vi "UT_Cognex.vi"() -> ()   [LabVIEW 2019, in "Kolmogan Library 1.lvlib"]
uses:
  Kolmogan Library 1.lvlib
panel:
  out "current time 5":timestamp
  out "指示燈":bool
  out "current time":timestamp
  out "Data":string
  out "Final result":string
  out "Trigger Success":bool
  out "螺絲檢測結果":string="檢測完成"
  out "右邊結果":string
  out "左邊結果":string
  out "檢測結果R":bool
  out "檢測結果L":bool
  out "R array":sgl[][](array[numeric])
  out "L array":sgl[][](array[numeric])
  out "掃高度次數":i32
  out "End time 4":timestamp=timestamp(3742957067.58093 s since 1904-01-01)
  out "移動完成 4":bool=TRUE
  out "Error status 4":bool
  out "等候逾時 4":bool
  out "剩餘秒數 4":i32=5
  in  "等候秒數 4":i32=40
  out "current time 4":timestamp=timestamp(3742957049.546739 s since 1904-01-01)
  out "找到原點":bool=TRUE
  in  "Trigger":u16(ring) items=["等待觸發", "觸發拍攝"]
  out "current time 3":timestamp=timestamp(3742956976.4306865 s since 1904-01-01)
  out "剩餘秒數 3":i32=9
  out "等候逾時 3":bool
  out "Error status 3":bool
  out "移動完成 3":bool=TRUE
  out "Motion State":bool[](array[boolean])=[FALSE, TRUE, TRUE, FALSE, FALSE, FALSE, FALSE, FALSE, FALSE, FALSE, FALSE, TRUE, FALSE, FALSE, FALSE, TRUE, FALSE, FALSE, FALSE, FALSE, FALSE, FALSE, FALSE, FALSE, FALSE, FALSE, FALSE, FALSE, FALSE, FALSE, FALSE, FALSE]
  in  "等候秒數 3":i32=15
  out "current time 2":timestamp=timestamp(3742956973.4187617 s since 1904-01-01)
  out "Error status 2":bool
  out "等候逾時 2":bool
  out "剩餘秒數 2":i32=5
  in  "等候秒數 2":i32=15
  out "State machine":i32=4
  out "等待觸發":bool=TRUE
  out "Offset array":dbl[](array[numeric])
  out "分析計算delay":u32=100
  out "使用流程":bool
  out "螺絲高度LL":dbl=2.1 format="%#_13g"
  out "螺絲高度UL":dbl=2.4009
  out "txt path":path
  out "L_file":string
  out "R_file":string
  in  "D2502.1 螺絲檢測 Ready":bool=TRUE
  in  "D2610 螺絲檢測完成":i16
  out "error out 2":errorcluster
  out "指令結果":string
  out "等待指令":string
  out "密碼":string
  out "帳號":string
  out "error out":errorcluster
  out "Success":bool
  in  "選項二: 觸發":bool
  in  "選項一: 監聽結果":bool
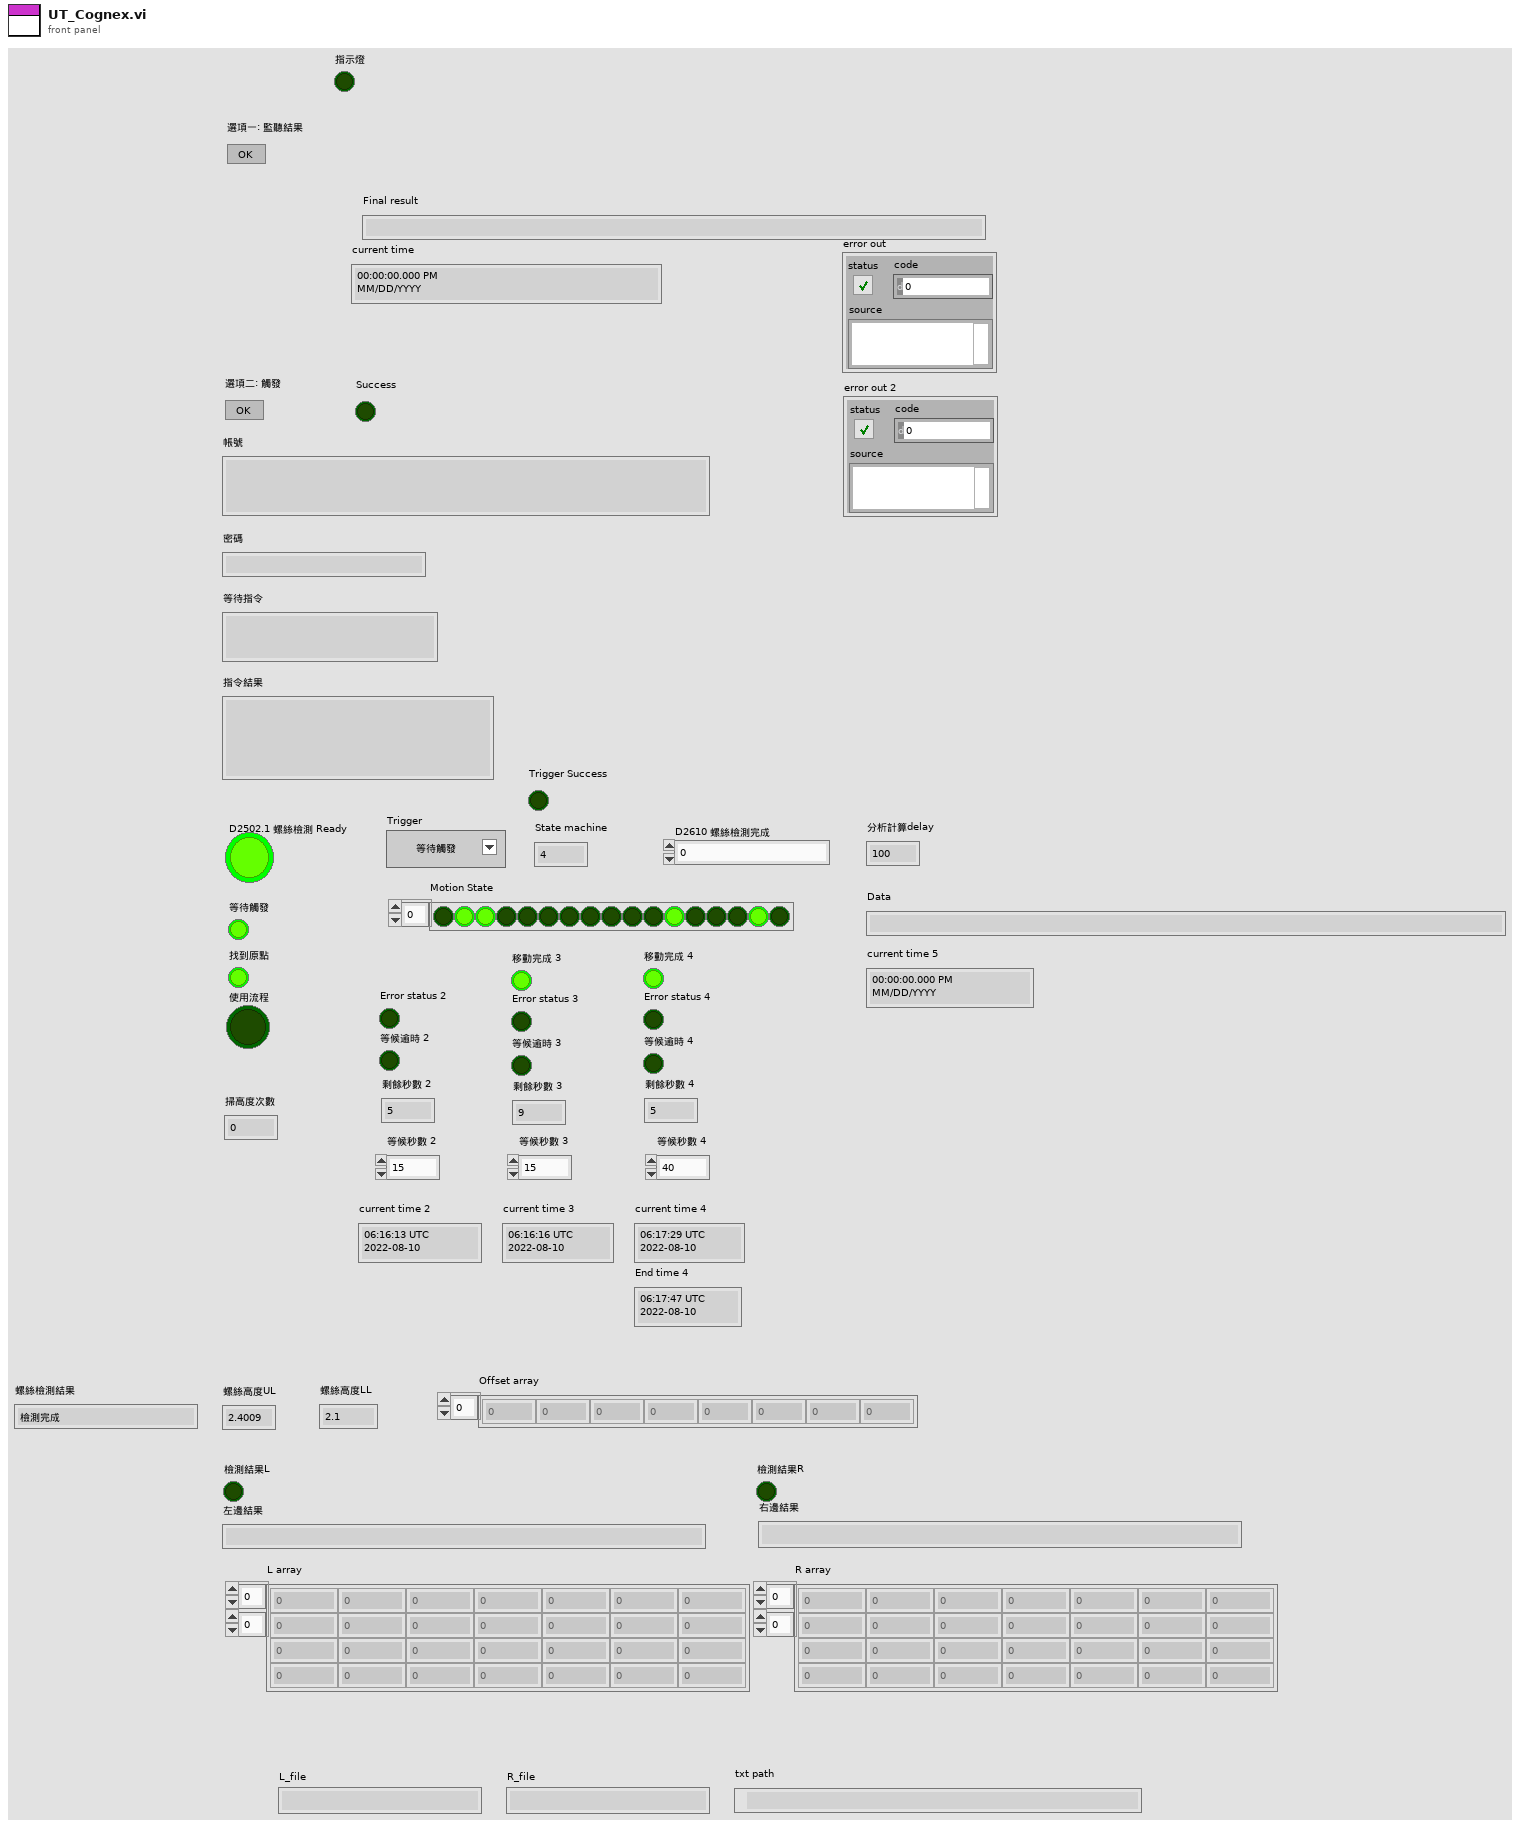
[diagram p1: front panel]
types:
  T1 = cluster{"sh_1":dbl, "sh_2":dbl, "sh_3":dbl, "sh_4":dbl, "sh_5":dbl, "sh_6":dbl}
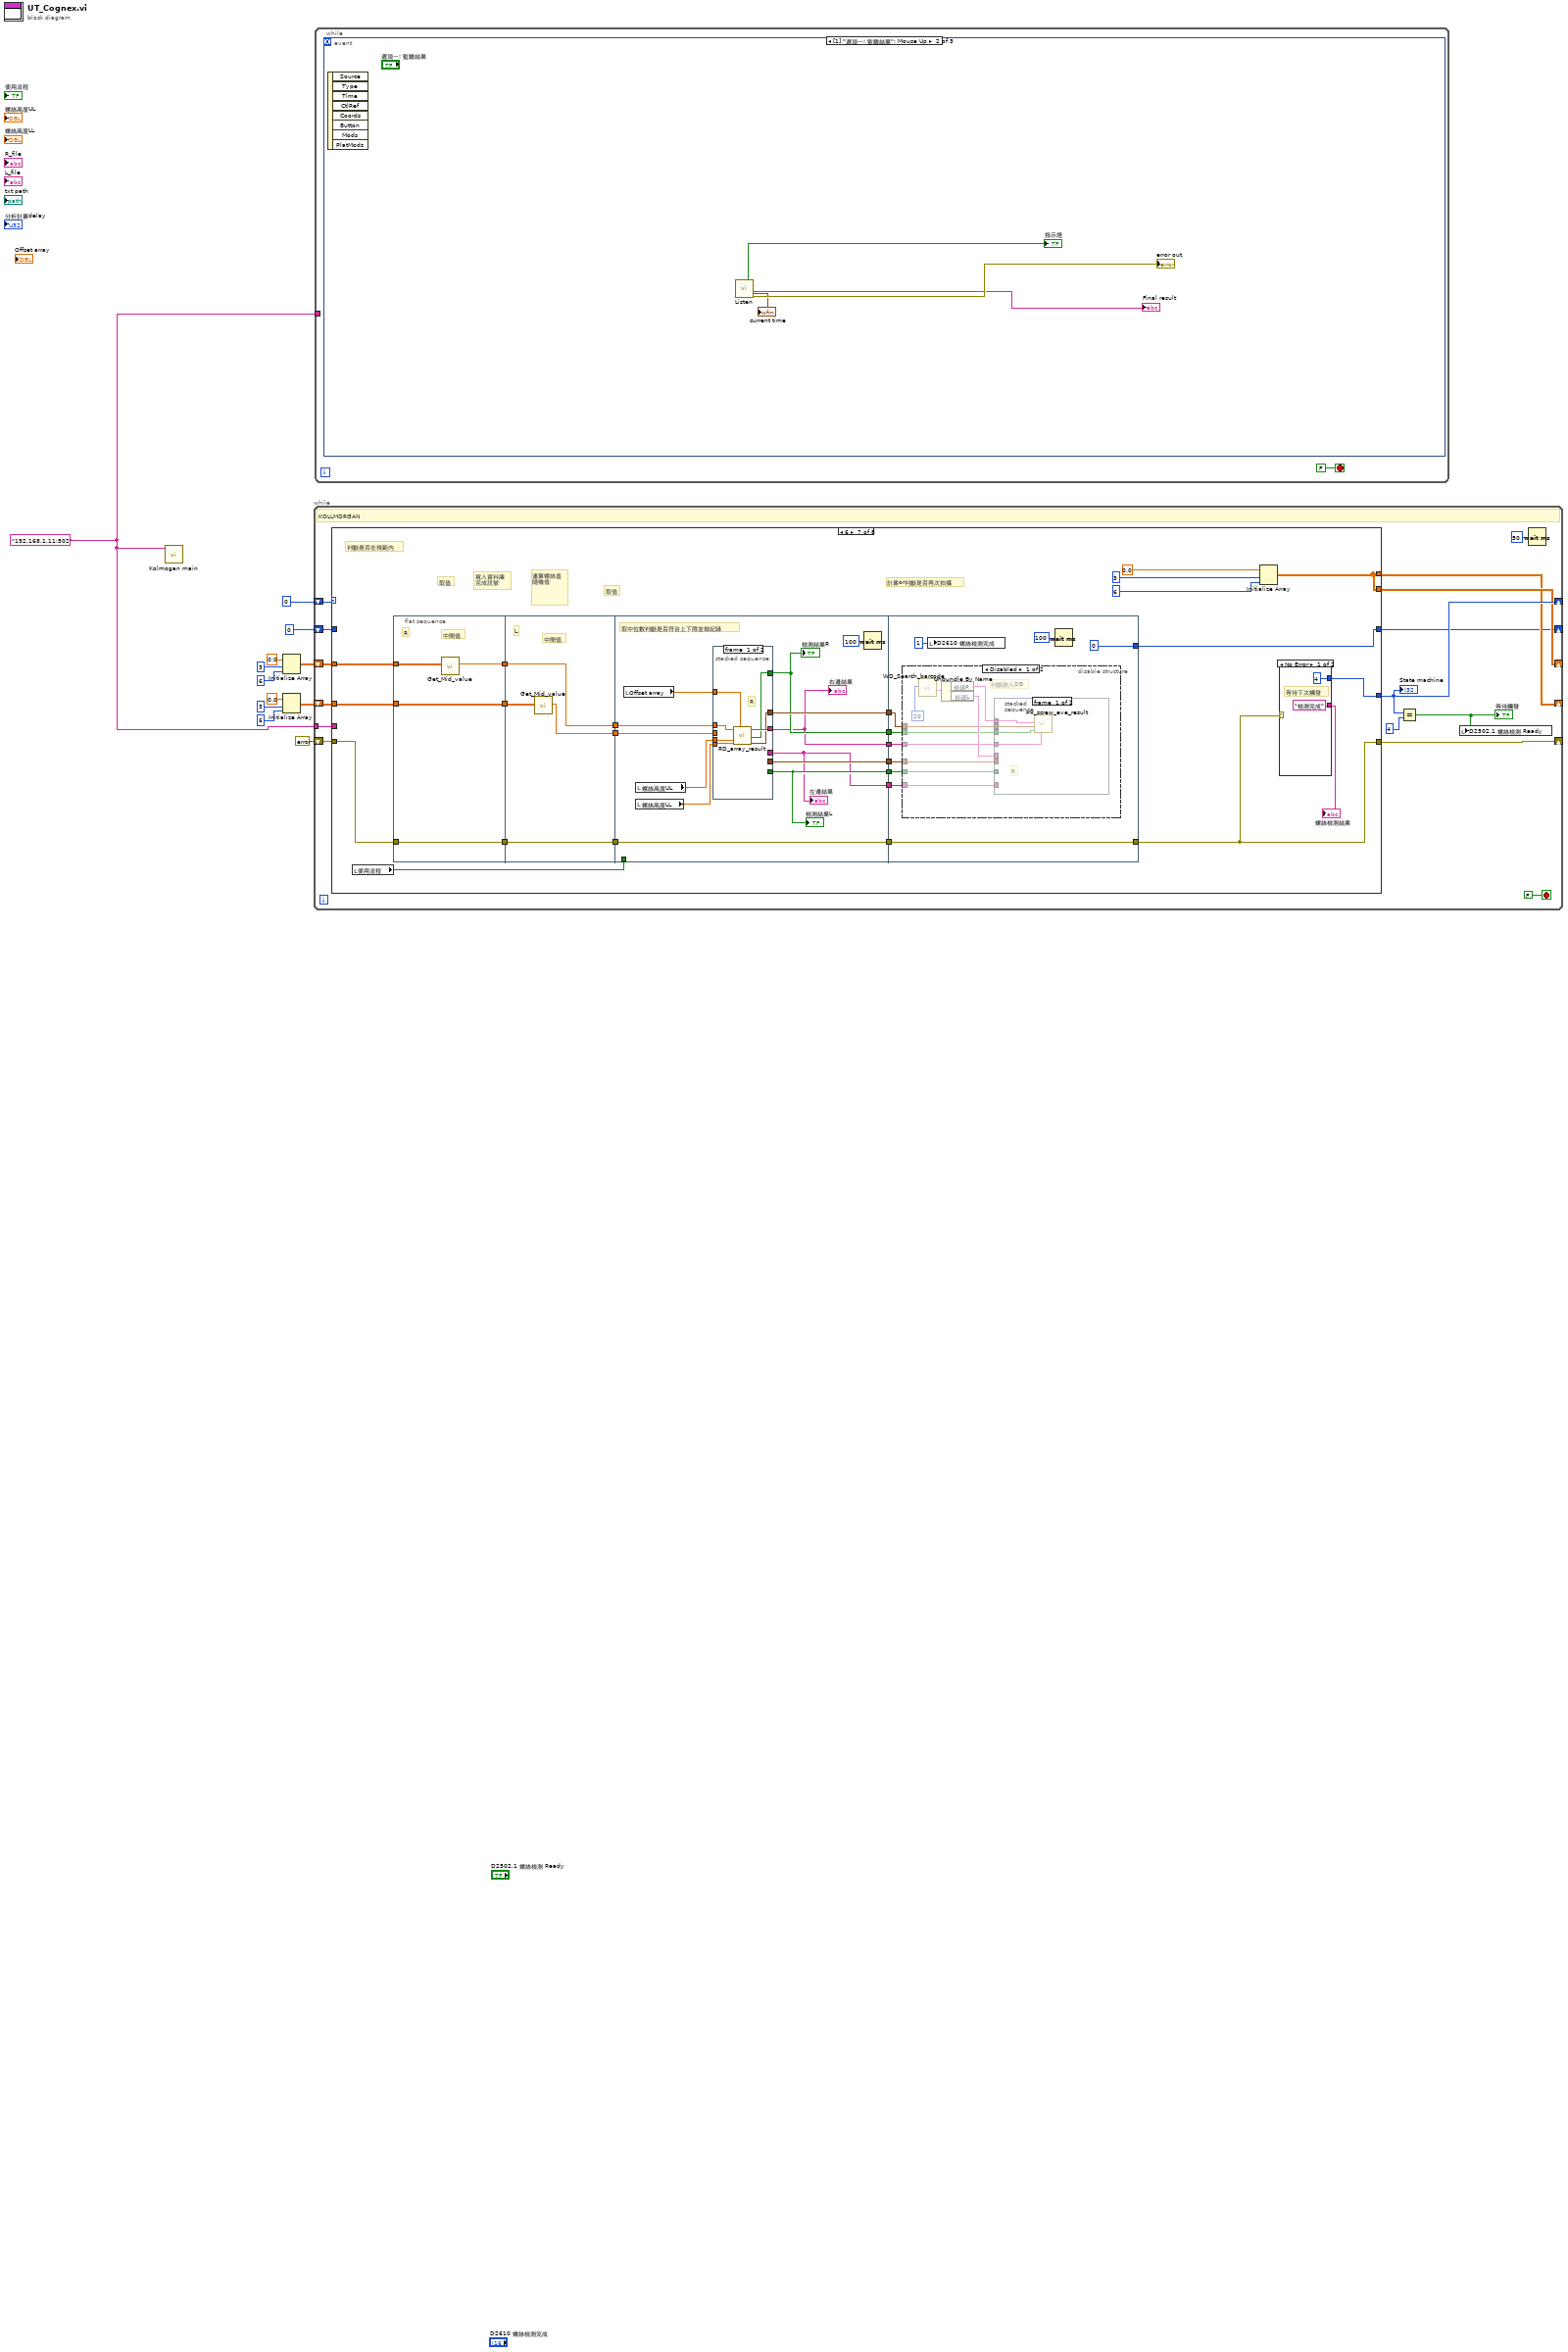
[diagram p0: block diagram]
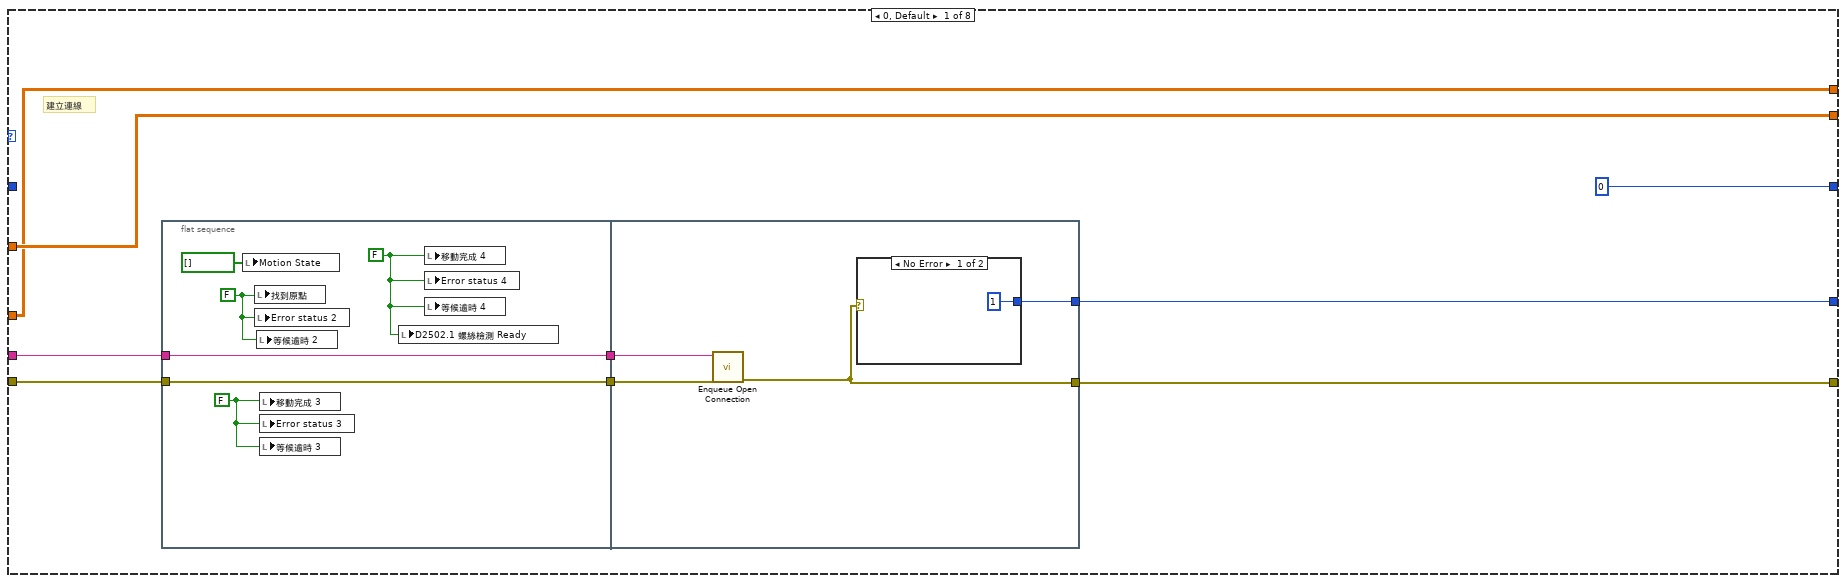
[diagram p2: hidden frame]
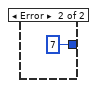
[diagram p3: hidden frame]
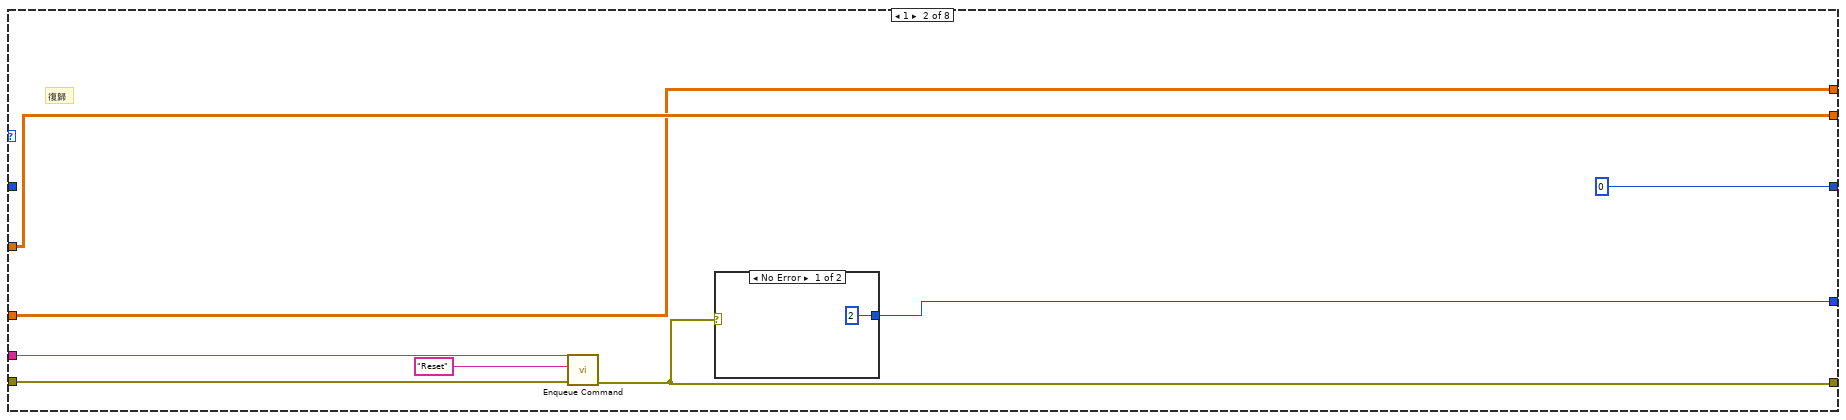
[diagram p4: hidden frame]
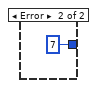
[diagram p5: hidden frame]
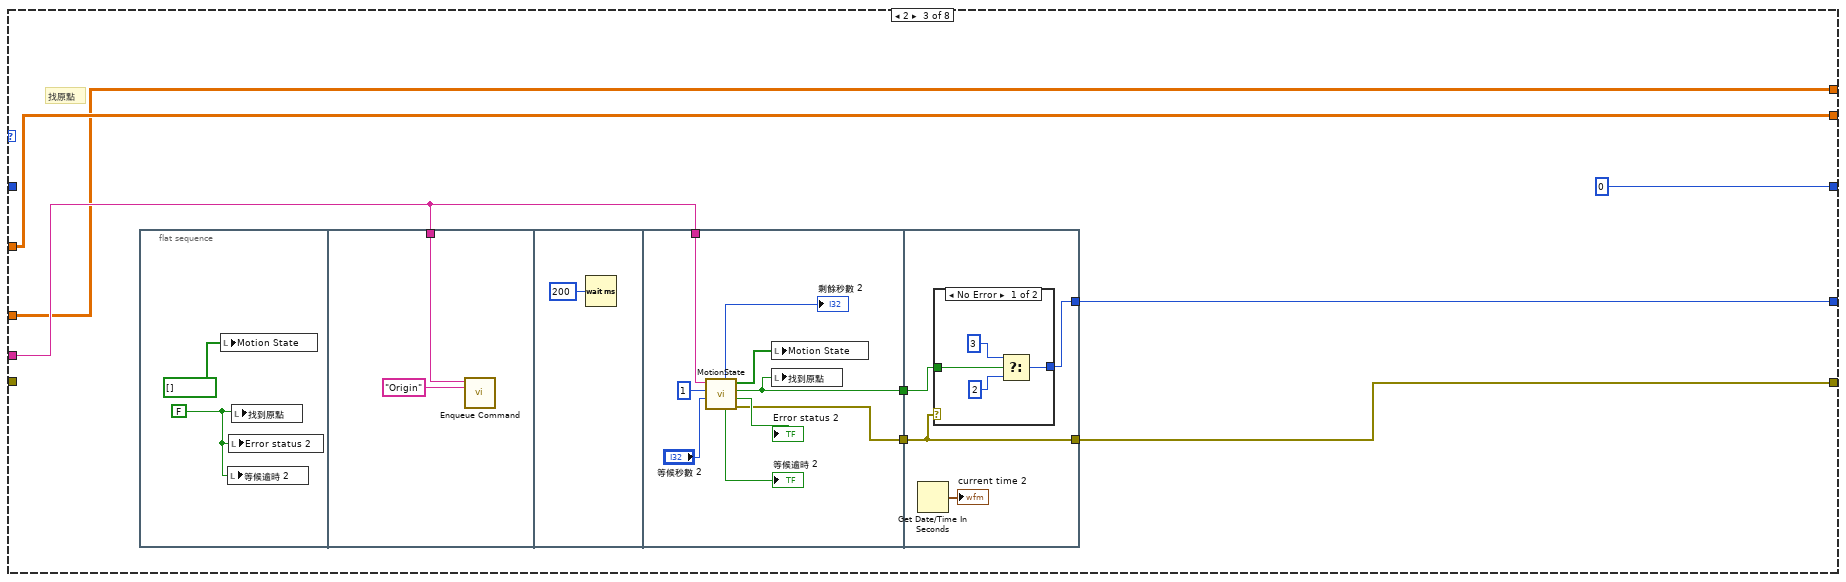
[diagram p6: hidden frame]
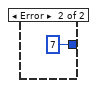
[diagram p7: hidden frame]
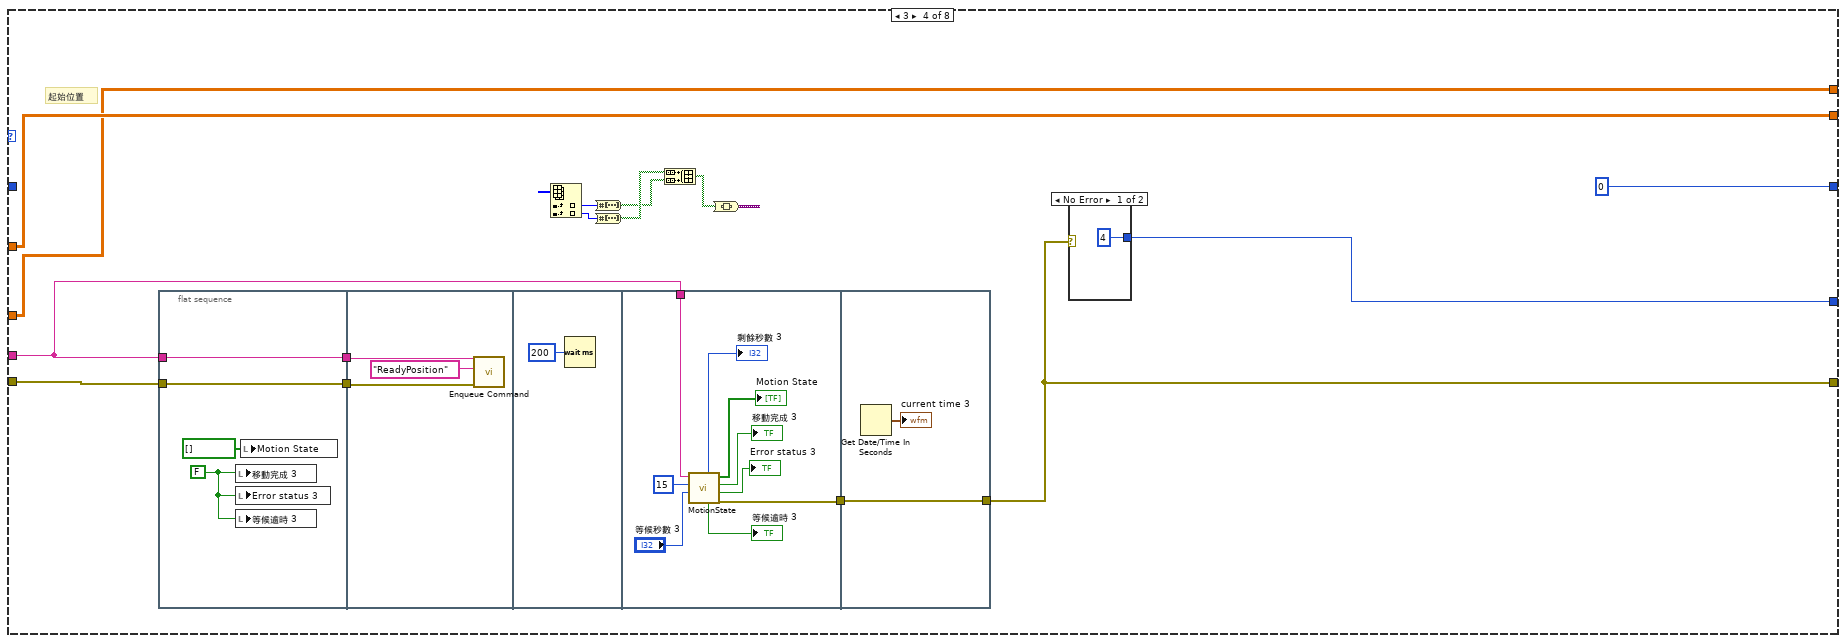
[diagram p8: hidden frame]
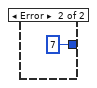
[diagram p9: hidden frame]
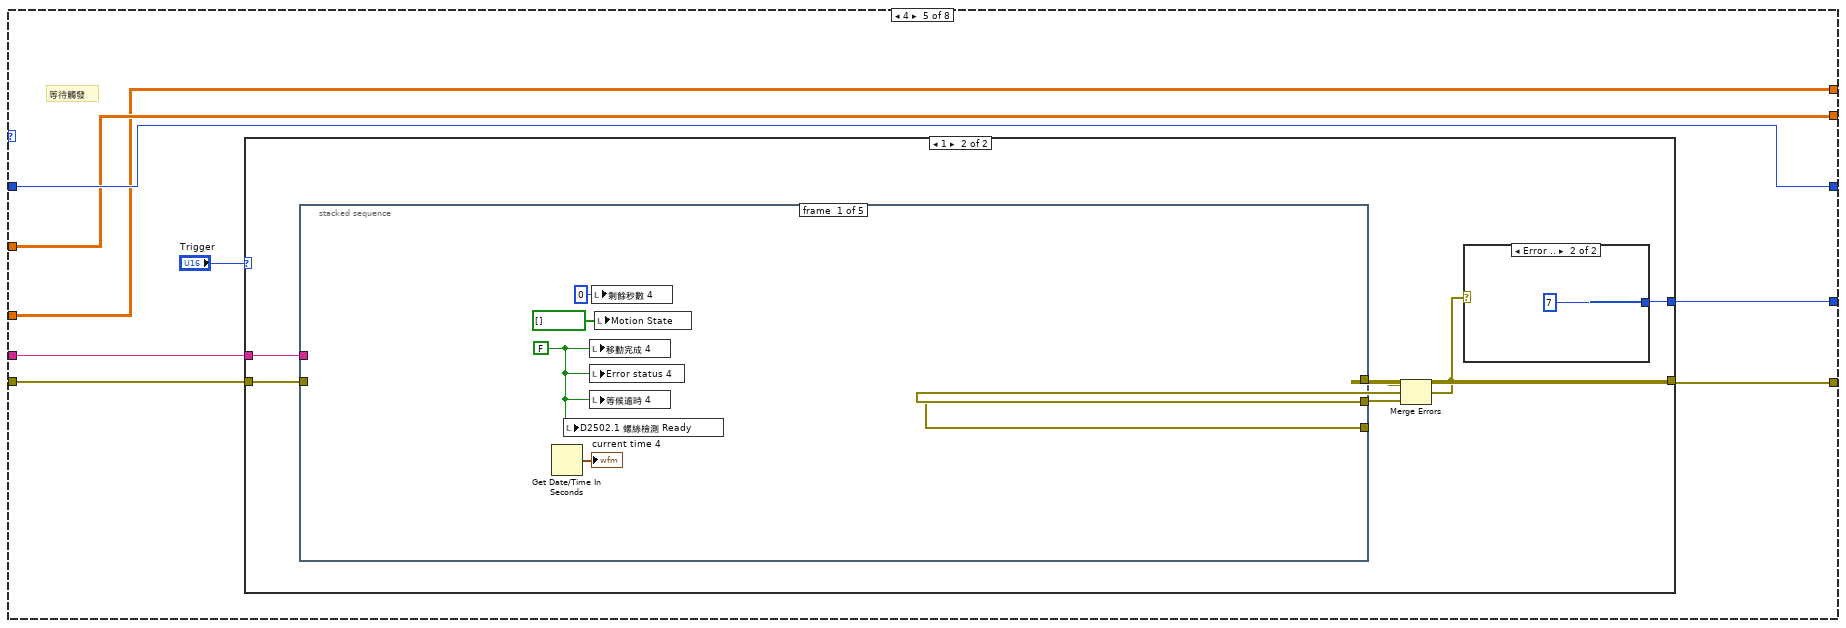
[diagram p10: hidden frame]
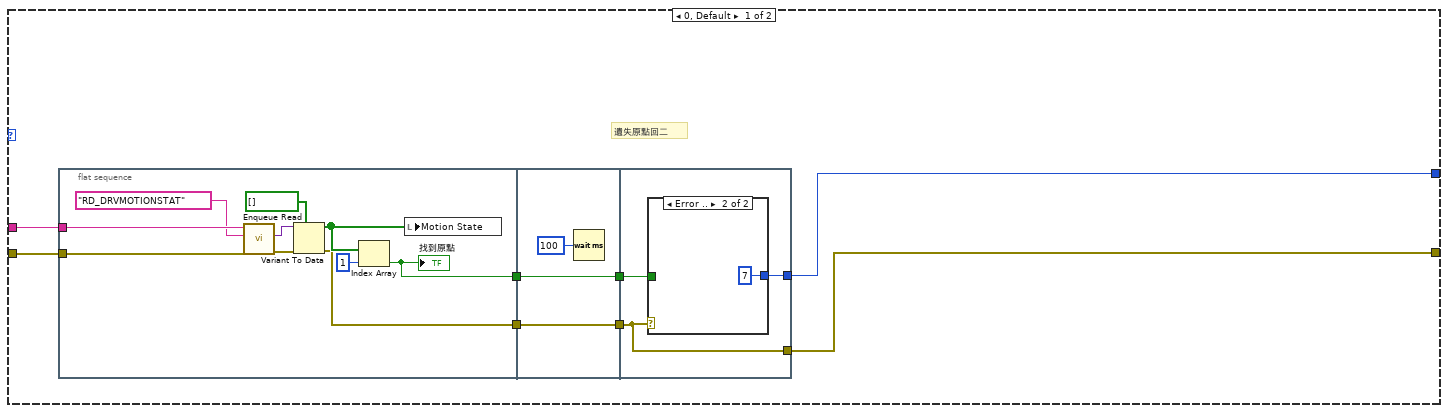
[diagram p11: hidden frame]
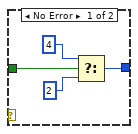
[diagram p12: hidden frame]
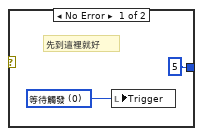
[diagram p13: hidden frame]
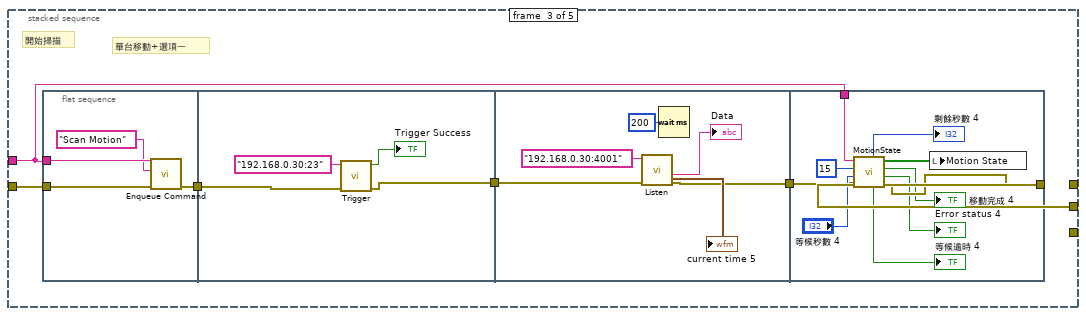
[diagram p15: hidden frame]
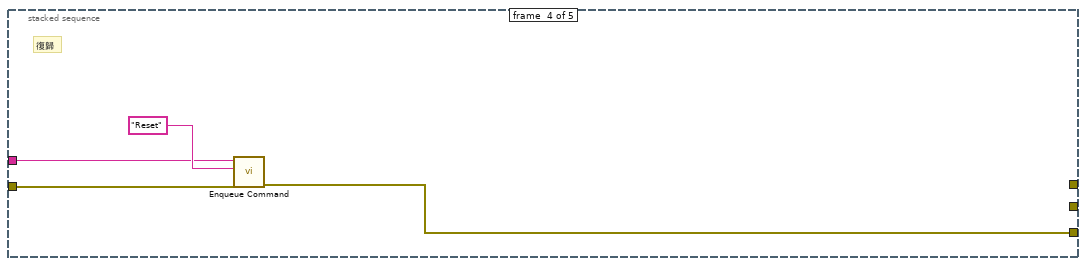
[diagram p16: hidden frame]
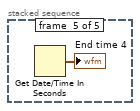
[diagram p17: hidden frame]
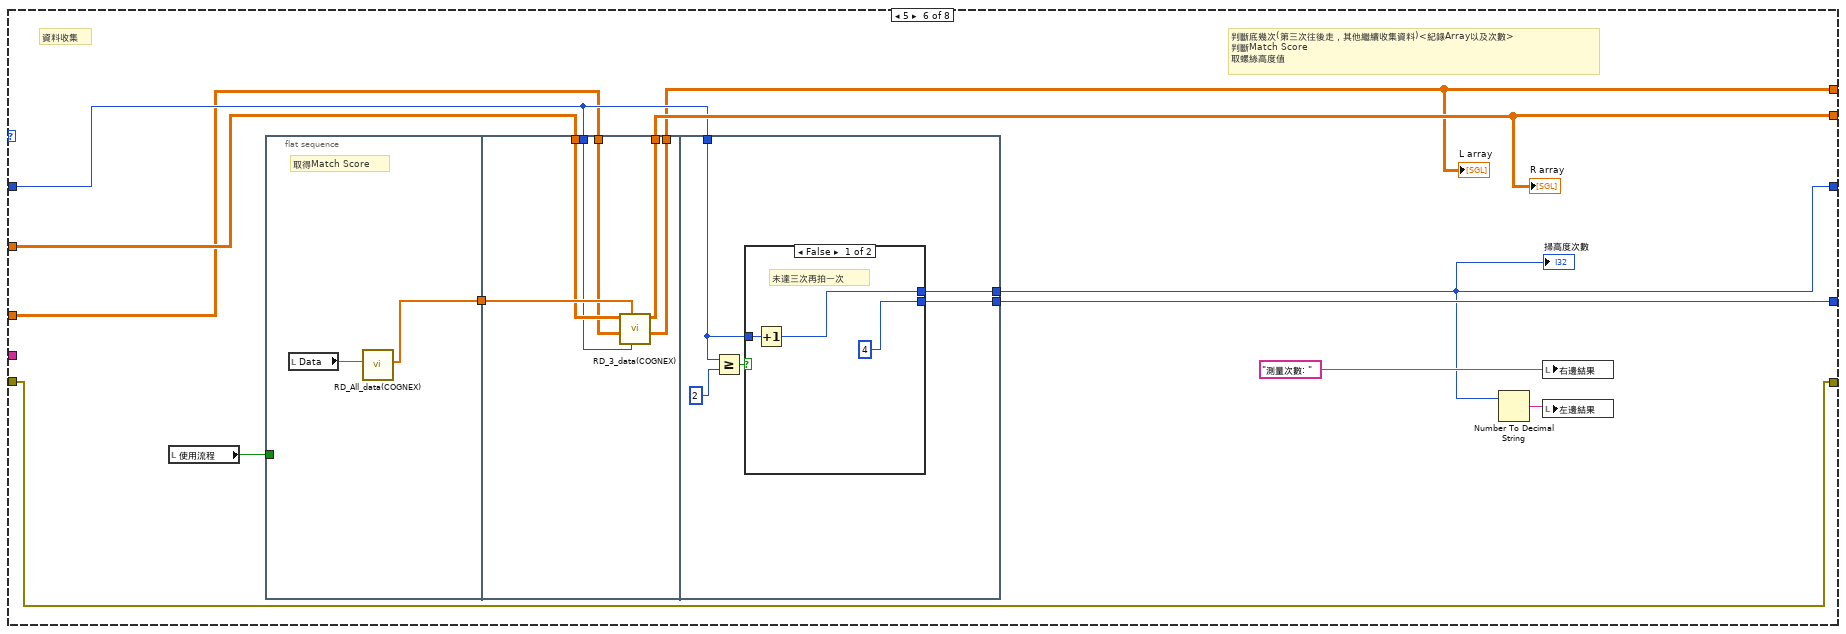
[diagram p18: hidden frame]
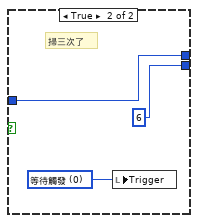
[diagram p19: hidden frame]
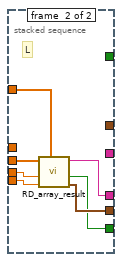
[diagram p20: hidden frame]
diagram:
  w1 = "192.168.1.11:502" ("Name")
  n1 = call "Kolmogan main.vi"("Name"=w1) -> ()  [unwired: 10 in, 1 out]
  n2 = Initialize Array(sgl 0.0 ("element"), 3 ("dimension size"), 6 ("dimension size")) -> (w6:sgl[][])
  n3 = Initialize Array(sgl 0.0 ("element"), 3 ("dimension size"), 6 ("dimension size")) -> (w2:sgl[][])
  n4 = while {
    shift-right: [w26] -> _
    shift-left: errorcluster {"status"=FALSE, "code"=0, "source"=""} ("Error Out") -> [w25]
    shift-right: [w23] -> _
    shift-left: 0 -> [w27]
    tunnel: w1 -> [w20]
    shift-right: [w13] -> _
    shift-left: 0 -> [w18]
    shift-right: [w16] -> _
    shift-left: w6 -> [w17]
    shift-right: [w14] -> _
    shift-left: w2 -> [w15]
    stop <- FALSE stop-if-true
    # "KOLLMORGAN"
    n5 = case shown="6" w27 {
      tunnel: w20 -> [w36 w54 w66 w97 w126 _ _ w336]
      tunnel: [w34 w53 w65 w96 w124 w214 w260 w337] -> w26
      tunnel: w25 -> [w35 w55 _ w99 w125 w214 w261 w338]
      tunnel: [w33 w52 w62 w98 w127 w215 w262 w339] -> w23
      tunnel: w18 -> [_ _ _ _ w123 w216 _ _]
      tunnel: w17 -> [w29 w50 w60 w91 w122 w218 w255 _]
      tunnel: [w29 w50 w60 w91 w122 w217 w241 w331] -> w16
      tunnel: w15 -> [w28 w49 w59 w90 w121 w209 w254 _]
      tunnel: [w28 w49 w59 w90 w121 w208 w241 w331] -> w14
      tunnel: [0 0 0 0 w123 w211 w245 0] -> w13
      frame 0, Default {
        # "建立連線"
        n6 = flat-sequence {
          tunnel: w35 -> [w41]
          tunnel: w36 -> [w42]
          tunnel: [w42] -> w32
          tunnel: [w41] -> w31
          tunnel: [w44] -> w34
          tunnel: [w43] -> w33
          tunnel: w32 -> [w46]
          tunnel: w31 -> [w45]
          frame #0 {
            w37 = FALSE ("移動完成")
            w38 = FALSE ("移動完成")
            w39 = FALSE ("移動完成")
            n7 = local write "Motion State"(bool[] [] ("Motion State")) -> ()
            n8 = local write "找到原點"(w39) -> ()
            n9 = local write "Error status 2"(w39) -> ()
            n10 = local write "等候逾時 2"(w39) -> ()
            n11 = local write "移動完成 3"(w38) -> ()
            n12 = local write "Error status 3"(w38) -> ()
            n13 = local write "等候逾時 3"(w38) -> ()
            n14 = local write "D2502.1 螺絲檢測 Ready"(w37) -> ()
            n15 = local write "移動完成 4"(w37) -> ()
            n16 = local write "Error status 4"(w37) -> ()
            n17 = local write "等候逾時 4"(w37) -> ()
          }
          frame #1 {
            n18 = call "Enqueue Open Connection.vi"("Error In"=w45, "Name"=w46) -> ("Error Out"=w44:errorcluster)  [unwired: 9 in]
            n19 = case shown="No Error" w44 {
              tunnel: [1 7] -> w43
              frame No Error {
              }
              frame Error {
              }
            }
          }
        }
      }
      frame 1 {
        # "復歸"
        n20 = call "Enqueue Command.vi"("Error In"=w55, "Message"="Reset", "Name"=w54) -> ("Error Out"=w53:errorcluster)  [unwired: 8 in]
        n21 = case shown="No Error" w53 {
          tunnel: [2 7] -> w52
          frame No Error {
          }
          frame Error {
          }
        }
      }
      frame 2 {
        # "找原點"
        n22 = flat-sequence {
          tunnel: w66 -> [w70]
          tunnel: w66 -> [w78]
          tunnel: [w73] -> w64
          tunnel: [w72] -> w63
          tunnel: [w81] -> w65
          tunnel: w64 -> [w81]
          tunnel: w63 -> [w83]
          tunnel: [w82] -> w62
          frame #0 {
            w68 = FALSE ("移動完成")
            n23 = local write "Motion State"(bool[] [] ("Motion State")) -> ()
            n24 = local write "等候逾時 2"(w68) -> ()
            n25 = local write "Error status 2"(w68) -> ()
            n26 = local write "找到原點"(w68) -> ()
          }
          frame #1 {
            n27 = call "Enqueue Command.vi"("Message"="Origin", "Name"=w70) -> ()  [unwired: 9 in, 1 out]
          }
          frame #2 {
            n28 = Wait (ms)(milliseconds to wait=u32 200) -> ()  [unwired: 1 out]
          }
          frame #3 {
            n29 = call "MotionState.vi"("等候秒數"="等候秒數 2", "index"=1, "IP:Port"=w78) -> ("error out"=w73:errorcluster, "Error status"=→"Error status 2":bool, "移動完成"=w72:bool, "Motion State"=w77:bool[], "等候逾時"=→"等候逾時 2":bool, "剩餘秒數"=→"剩餘秒數 2":i32)  [unwired: 3 in]
            n30 = local write "Motion State"(w77) -> ()
            n31 = local write "找到原點"(w72) -> ()
          }
          frame #4 {
            n32 = Get Date/Time In Seconds() -> (seconds since 1Jan1904=→"current time 2":timestamp)
            n33 = case shown="No Error" w81 {
              tunnel: w83 -> [w88 _]
              tunnel: [w85 7 ("f")] -> w82
              frame No Error {
                n34 = Select(t=3, s=w88, f=2) -> (s? t:f=w85:i32)
              }
              frame Error {
              }
            }
          }
        }
      }
      frame 3 {
        # "起始位置"
        n35 = flat-sequence {
          tunnel: w97 -> [w102]
          tunnel: w99 -> [w103]
          tunnel: [w103] -> w95
          tunnel: [w102] -> w94
          tunnel: w95 -> [w105]
          tunnel: w94 -> [w104]
          tunnel: w97 -> [w116]
          tunnel: [w115] -> w93
          tunnel: [w118] -> w96
          tunnel: w93 -> [w118]
          frame #0 {
            w100 = FALSE ("移動完成")
            n36 = local write "移動完成 3"(w100) -> ()
            n37 = local write "Error status 3"(w100) -> ()
            n38 = local write "等候逾時 3"(w100) -> ()
            n39 = local write "Motion State"(bool[] [] ("Motion State")) -> ()
          }
          frame #1 {
            n40 = call "Enqueue Command.vi"("Error In"=w105, "Message"="ReadyPosition", "Name"=w104) -> ()  [unwired: 8 in, 1 out]
          }
          frame #2 {
            n41 = Wait (ms)(milliseconds to wait=u32 200) -> ()  [unwired: 1 out]
          }
          frame #3 {
            n42 = call "MotionState.vi"("等候秒數"="等候秒數 3", "index"=15, "IP:Port"=w116) -> ("error out"=w115:errorcluster, "Error status"=→"Error status 3":bool, "移動完成"=→"移動完成 3":bool, "Motion State"=→"Motion State":bool[], "等候逾時"=→"等候逾時 3":bool, "剩餘秒數"=→"剩餘秒數 3":i32)  [unwired: 3 in]
          }
          frame #4 {
            n43 = Get Date/Time In Seconds() -> (seconds since 1Jan1904=→"current time 3":timestamp)
          }
        }
        n44 = case shown="No Error" w96 {
          tunnel: [4 7] -> w98
          frame No Error {
          }
          frame Error {
          }
        }
      }
      frame 4 {
        # "等待觸發"
        n45 = case shown="1" "Trigger" {
          tunnel: [w133 w159] -> w127
          tunnel: w126 -> [w136 w164]
          tunnel: w125 -> [w129 w163]
          tunnel: [w130 w158] -> w124
          frame 0, Default {
            # "遺失原點回二"
            n46 = flat-sequence {
              tunnel: w136 -> [w146]
              tunnel: [w139] -> w134
              tunnel: [w138] -> w131
              tunnel: w129 -> [w137]
              tunnel: [w148] -> w135
              tunnel: w134 -> [w148]
              tunnel: [w147] -> w132
              tunnel: w131 -> [w147]
              tunnel: w135 -> [w152]
              tunnel: [w151] -> w133
              tunnel: w132 -> [w150]
              tunnel: [w150] -> w130
              frame #0 {
                n47 = call "Enqueue Read.vi"("Error In"=w137, "Message"="RD_DRVMOTIONSTAT", "Name"=w146) -> ("Error Out"=w144:errorcluster, "Data"=w143:variant)  [unwired: 7 in]
                n48 = Variant To Data(error in=w144, type=bool[] [] ("appended array"), Variant=w143) -> (data=w140:bool[], error out=w138:errorcluster)
                n49 = Index Array(array=w140, index=1) -> (element=w139:bool)
                "找到原點" <- w139
                n50 = local write "Motion State"(w140) -> ()
              }
              frame #1 {
                n51 = Wait (ms)(milliseconds to wait=u32 100) -> ()  [unwired: 1 out]
              }
              frame #2 {
                n52 = case shown="Error .." w150 {
                  tunnel: w152 -> [w156 _]
                  tunnel: [w153 7 ("f")] -> w151
                  frame No Error {
                    n53 = Select(t=4, s=w156, f=2) -> (s? t:f=w153:i32)
                  }
                  frame Error {
                  }
                }
              }
            }
          }
          frame 1 {
            n54 = stacked-sequence {
              tunnel: w164 -> [_ _ w177 w205 _]
              tunnel: w163 -> [_ w172 w178 w204 _]
              tunnel: [_ w172 _ _ _] -> w162
              tunnel: [_ _ w176 _ _] -> w161
              tunnel: [_ _ _ w203 _] -> w160
              frame #0 {
                w168 = FALSE ("移動完成")
                n55 = Get Date/Time In Seconds() -> (seconds since 1Jan1904=→"current time 4":timestamp)
                n56 = local write "D2502.1 螺絲檢測 Ready"(w168) -> ()
                n57 = local write "移動完成 4"(w168) -> ()
                n58 = local write "Error status 4"(w168) -> ()
                n59 = local write "等候逾時 4"(w168) -> ()
                n60 = local write "剩餘秒數 4"(0 ("剩餘秒數")) -> ()
                n61 = local write "Motion State"(bool[] [] ("Motion State")) -> ()
              }
              frame #1 {
                # "選項一"
                # "相機開啟"
              }
              frame #2 {
                # "華台移動+選項一"
                # "開始掃描"
                n62 = flat-sequence {
                  tunnel: w178 -> [w182]
                  tunnel: w177 -> [w181]
                  tunnel: [w179] -> w175
                  tunnel: w175 -> [w185]
                  tunnel: [w183] -> w174
                  tunnel: w174 -> [w188]
                  tunnel: [w187] -> w173
                  tunnel: w177 -> [w202]
                  tunnel: [w200] -> w176
                  tunnel: w173 -> [w193]
                  frame #0 {
                    n63 = call "Enqueue Command.vi"("Error In"=w182, "Message"="Scan Motion", "Name"=w181) -> ("Error Out"=w179:errorcluster)  [unwired: 8 in]
                  }
                  frame #1 {
                    n64 = call "Trigger.vi"("error in (no error)"=w185, "COGNEX IP:PORT(CMD)"="192.168.0.30:23") -> ("error out"=w183:errorcluster, "Success"=→"Trigger Success":bool)  [unwired: 4 in, 4 out]
                  }
                  frame #2 {
                    n65 = call "Listen.vi"("error in (no error)"=w188, "COGNEX IP:Port(recv)"="192.168.0.30:4001") -> ("error out"=w187:errorcluster, "f"=→"Data":string, "current time"=→"current time 5":timestamp)  [unwired: 4 in, 3 out]
                    n66 = Wait (ms)(milliseconds to wait=u32 200) -> ()  [unwired: 1 out]
                  }
                  frame #3 {
                    n67 = call "MotionState.vi"("Error In"=w193, "等候秒數"="等候秒數 4", "index"=15, "IP:Port"=w202) -> ("error out"=w200:errorcluster, "Error status"=→"Error status 4":bool, "移動完成"=→"移動完成 4":bool, "Motion State"=w201:bool[], "等候逾時"=→"等候逾時 4":bool, "剩餘秒數"=→"剩餘秒數 4":i32)  [unwired: 2 in]
                    n68 = local write "Motion State"(w201) -> ()
                  }
                }
              }
              frame #3 {
                # "復歸"
                n69 = call "Enqueue Command.vi"("Error In"=w204, "Message"="Reset", "Name"=w205) -> ("Error Out"=w203:errorcluster)  [unwired: 8 in]
              }
              frame #4 {
                n70 = Get Date/Time In Seconds() -> (seconds since 1Jan1904=→"End time 4":timestamp)
              }
            }
            n71 = Merge Errors(w162, w161, w160) -> (w158:errorcluster)
            n72 = case shown="Error .." w158 {
              tunnel: [5 7] -> w159
              frame No Error {
                w165 = u16 0 items=["等待觸發", "觸發拍攝"] ("Menu Ring")
                # "先到這裡就好"
                n73 = local write "Trigger"(w165) -> ()
              }
              frame Error {
              }
            }
          }
        }
      }
      frame 5 {
        # "資料收集"
        # "判斷底幾次(第三次往後走，其他繼續收集資料)<紀錄Array以及次數>\n判斷Match Score\n取螺絲高度值"
        n74 = local read "使用流程"() -> (w219:bool)
        n75 = flat-sequence {
          tunnel: w219 -> [_]
          tunnel: [w220] -> w210
          tunnel: w218 -> [w226]
          tunnel: w216 -> [w222]
          tunnel: [w225] -> w217
          tunnel: w210 -> [w227]
          tunnel: w209 -> [w224]
          tunnel: [w223] -> w208
          tunnel: w216 -> [w229]
          tunnel: [w230] -> w215
          tunnel: [w228] -> w211
          frame #0 {
            # "取得Match Score"
            n76 = local read "Data"() -> (w221:string)
            n77 = call "RD_All_data(COGNEX).vi"("Dara"=w221) -> ("Array"=w220:dbl[])  [unwired: 10 in]
          }
          frame #1 {
            n78 = call "RD_3_data(COGNEX).vi"("index (row)"=w222, "Array"=w227, "Data array 2"=w224, "Data array"=w226) -> ("output array 2"=w223:sgl[][], "output array"=w225:sgl[][])  [unwired: 6 in]
          }
          frame #2 {
            n79 = Greater Or Equal?(x=w229, y=2) -> (x >= y?=w231:bool)
            n80 = case shown="False" w231 {
              tunnel: [4 ("f") 6 ("f")] -> w230
              tunnel: w229 -> [w234 w237]
              tunnel: [w233 w237] -> w228
              frame False {
                # "未達三次再拍一次"
                n81 = Increment(x=w234) -> (x+1=w233:i32)
              }
              frame True {
                w236 = u16 0 items=["等待觸發", "觸發拍攝"] ("Menu Ring")
                # "掃三次了"
                n82 = local write "Trigger"(w236) -> ()
              }
            }
          }
        }
        n83 = Number To Decimal String(number=w211) -> (decimal integer string=w213:string)  [unwired: 1 in]
        n84 = local write "右邊結果"("測量次數: " ("右邊結果")) -> ()
        n85 = local write "左邊結果"(w213) -> ()
        "R array" <- w217
        "L array" <- w208
        "掃高度次數" <- w211
      }
      frame 6 {
        # "判斷是否在規範內"
        # "計算or判斷是否再次拍攝"
        # "取值"
        # "運算螺絲直\n隨機值"
        # "寫入資料庫\n完成訊號"
        # "取值"
        n86 = local read "使用流程"() -> (w257:bool)
        n87 = flat-sequence {
          tunnel: w261 -> [w267]
          tunnel: [w267] -> w256
          tunnel: w255 -> [w266]
          tunnel: w254 -> [w265]
          tunnel: [w265] -> w253
          tunnel: [w264] -> w251
          tunnel: [w271] -> w259
          tunnel: w256 -> [w271]
          tunnel: w253 -> [w270]
          tunnel: [w269] -> w252
          tunnel: w251 -> [w269]
          tunnel: [w268] -> w249
          tunnel: [w284] -> w258
          tunnel: w259 -> [w284]
          tunnel: w257 -> [_]
          tunnel: w252 -> [w279]
          tunnel: [w278] -> w250
          tunnel: w249 -> [w277]
          tunnel: [w276] -> w248
          tunnel: [w275] -> w247
          tunnel: [w274] -> w246
          tunnel: [w273] -> w240
          tunnel: [w272] -> w239
          tunnel: [w308] -> w260
          tunnel: w258 -> [w308]
          tunnel: w250 -> [w305]
          tunnel: w248 -> [w304]
          tunnel: w247 -> [w303]
          tunnel: w246 -> [w302]
          tunnel: [0] -> w245
          tunnel: w240 -> [w300]
          tunnel: w239 -> [w299]
          frame #0 {
            # "中間值"
            # "R"
            n88 = call "Get_Mid_value.vi"("Data array"=w266) -> ("Output"=w264:dbl[])  [unwired: 10 in]
          }
          frame #1 {
            # "中間值"
            # "L"
            n89 = call "Get_Mid_value.vi"("Data array"=w270) -> ("Output"=w268:dbl[])  [unwired: 10 in]
          }
          frame #2 {
            # "取中位數判斷是否符合上下限並做紀錄"
            n90 = local read "Offset array"() -> (w280:dbl[])
            n91 = local read "螺絲高度UL"() -> (w282:dbl)
            n92 = local read "螺絲高度LL"() -> (w281:dbl)
            n93 = stacked-sequence {
              tunnel: w282 -> [w289 w297]
              tunnel: w281 -> [w288 w296]
              tunnel: w280 -> [w290 w295]
              tunnel: w279 -> [w291 _]
              tunnel: [w287 _] -> w272
              tunnel: [w286 _] -> w274
              tunnel: [w285 _] -> w278
              tunnel: w277 -> [_ w298]
              tunnel: [_ w294] -> w273
              tunnel: [_ w293] -> w276
              tunnel: [_ w292] -> w275
              frame #0 {
                # "R"
                n94 = call "RD_array_result.vi"("Offset array"=w290, "lower limit"=w288, "upper limit"=w289, "Input"=w291) -> ("data"=w285:T1, "結果"=w286:bool, "數據結果"=w287:string)  [unwired: 5 in]
              }
              frame #1 {
                # "L"
                n95 = call "RD_array_result.vi"("Offset array"=w295, "lower limit"=w296, "upper limit"=w297, "Input"=w298) -> ("data"=w293:T1, "結果"=w292:bool, "數據結果"=w294:string)  [unwired: 5 in]
              }
            }
            "右邊結果" <- w272
            "左邊結果" <- w273
            "檢測結果R" <- w274
            "檢測結果L" <- w275
            n96 = Wait (ms)(milliseconds to wait=u32 100) -> ()  [unwired: 1 out]
          }
          frame #3 {
            n97 = disable-structure shown="Disabled" {
              disable-tunnel: w305 -> [w314 _]
              disable-tunnel: w304 -> [w313 _]
              disable-tunnel: w303 -> [w312 _]
              disable-tunnel: w302 -> [w311 _]
              disable-tunnel: w300 -> [w310 _]
              disable-tunnel: w299 -> [w309 _]
              frame Disabled {
                # "判斷謝入DB"
                n98 = call "WD_Search_barcode.vi"("workplace_name_id"=i16 20) -> ("workplace_data"=w318:cluster{"條碼R":string, "條碼L":string})  [unwired: 7 in, 3 out]
                n99 = Unbundle By Name(w318) -> ("條碼R"=w316:string, "條碼L"=w315:string)
                n100 = stacked-sequence {
                  tunnel: w316 -> [w322 _]
                  tunnel: w315 -> [_ w326]
                  tunnel: w314 -> [w321 _]
                  tunnel: w313 -> [_ w325]
                  tunnel: w312 -> [_ w324]
                  tunnel: w311 -> [w320 _]
                  tunnel: w310 -> [_ w323]
                  tunnel: w309 -> [w319 _]
                  frame #0 {
                    # "R"
                    n101 = call "PR_screw_eve_result.vi"("結果"=w319, "result"=w320, "data"=w321, "barcode"=w322) -> ()  [unwired: 8 in]
                  }
                  frame #1 {
                    # "L"
                    n102 = call "PR_screw_eve_result.vi"("結果"=w323, "result"=w324, "data"=w325, "barcode"=w326) -> ()  [unwired: 8 in]
                  }
                }
              }
              frame Enabled {
              }
            }
            n103 = local write "D2610 螺絲檢測完成"(i16 1 ("D2610 螺絲檢測完成")) -> ()
            n104 = Wait (ms)(milliseconds to wait=u32 100) -> ()  [unwired: 1 out]
          }
        }
        n105 = Initialize Array(sgl 0.0 ("element"), 3 ("dimension size"), 6 ("dimension size")) -> (w241:sgl[][])
        n106 = case shown="No Error" w260 {
          tunnel: ["檢測完成" "Error 無結果"] -> w263
          tunnel: [4 7] -> w262
          frame No Error {
            # "等待下次觸發"
          }
          frame Error {
          }
        }
        "螺絲檢測結果" <- w263
      }
      frame 7 {
        n107 = disable-structure shown="Disabled" {
          disable-tunnel: _ -> [w341 _]
          disable-tunnel: w338 -> [w340 _]
          frame Disabled {
            n108 = case shown="Error .." w340 {
              selector: w340 -> [_ w346]
              tunnel: w341 -> [_ w342]
              frame No Error {
              }
              frame Error {
                n109 = Unbundle By Name(w346) -> ("code"=w345:i32, "source"=w343:string)
                n110 = Number To Decimal String(number=w345) -> (decimal integer string=w344:string)  [unwired: 1 in]
                n111 = call "Insert_Event_Log(classify)vi.vi"("classify"=i16 6, "data"=w343, "message"="Modbus通訊異常", "id"=w344, "DBlink"=w342) -> ()  [unwired: 6 in, 1 out]
              }
            }
          }
          frame Enabled {
          }
        }
        n112 = case shown="Error .." w338 {
          selector: w338 -> [w350 _]
          tunnel: [w350 w356] -> w337
          tunnel: [4 0] -> w339
          tunnel: w336 -> [_ w354]
          frame No Error {
          }
          frame Error {
            w351 = u16 0 items=["等待觸發", "觸發拍攝"] ("Menu Ring")
            n113 = call "Enqueue Close Connection.vi"("Name"=w354) -> ("Error Out"=w353:errorcluster)  [unwired: 10 in]
            n114 = call <vilib>:"Clear Errors.vi"("error in (no error)"=w353) -> ("error out"=w356:errorcluster)  [unwired: 5 in, 1 out]
            n115 = Wait (ms)(milliseconds to wait=u32 1000) -> ()  [unwired: 1 out]
            n116 = local write "D2610 螺絲檢測完成"(i16 1 ("D2610 螺絲檢測完成")) -> ()
            n117 = local write "Trigger"(w351) -> ()
          }
        }
        n118 = Initialize Array(sgl 0.0 ("element"), 3 ("dimension size"), 6 ("dimension size")) -> (w331:sgl[][])
      }
    }
    "State machine" <- w23
    n119 = Equal?(x=w23, y=4) -> (x = y?=w19:bool)
    "等待觸發" <- w19
    n120 = local write "D2502.1 螺絲檢測 Ready"(w19) -> ()
    n121 = Wait (ms)(milliseconds to wait=u32 50) -> ()  [unwired: 1 out]
  }
  n122 = while {
    tunnel: w1 -> [_]
    stop <- FALSE stop-if-true
    n123 = event shown="[1] \"選項一: 監聽結果\": Mouse Up" {
      selector: _ -> [_ _ _]
      dyn-events: _ -> [_ _ _]
      timeout: _ -> [_ _ _]
      event Timeout {
        n124 = event-data() -> ()  [unwired: 1 in, 3 out]
      }
      event "選項一: 監聽結果": Mouse Up {
        n125 = event-data() -> ()  [unwired: 1 in, 8 out]
        n126 = call "Listen.vi"() -> ("error out"=→"error out":errorcluster, "f"=→"Final result":string, "current time"=→"current time":timestamp, "指示燈"=→"指示燈":bool)  [unwired: 6 in, 2 out]
      }
      event "選項二: 觸發": Mouse Up {
        n127 = event-data() -> ()  [unwired: 1 in, 8 out]
        n128 = call "Trigger.vi"("error in (no error)"=errorcluster {"status"=FALSE, "code"=0, "source"=""}) -> ("error out"=→"error out 2":errorcluster, "密碼"=→"密碼":string, "等待指令"=→"等待指令":string, "Success"=→"Success":bool, "及時"=→"帳號":string, "指令結果"=→"指令結果":string)  [unwired: 5 in]
      }
    }
  }
